vi "Ex2_PagWeb.vi"(0 "WebBrowser":refnum<k7>(container), 8 "stop":bool, 11 "Web Page URL":string="http://") -> (3 "Web Page Title":string)   [LabVIEW 2020]
doc: "This example uses the Microsoft WebBrowser ActiveX control. It demonstrates how to register an ActiveX event callback and extract event data."
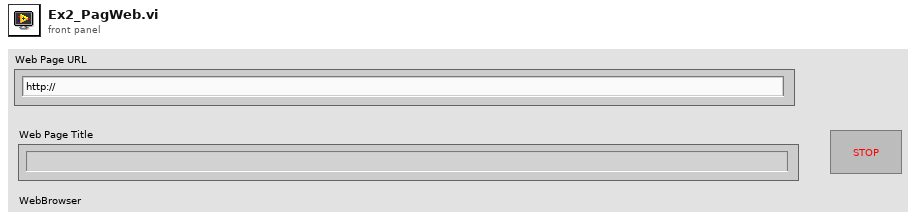
[diagram p1: front panel]
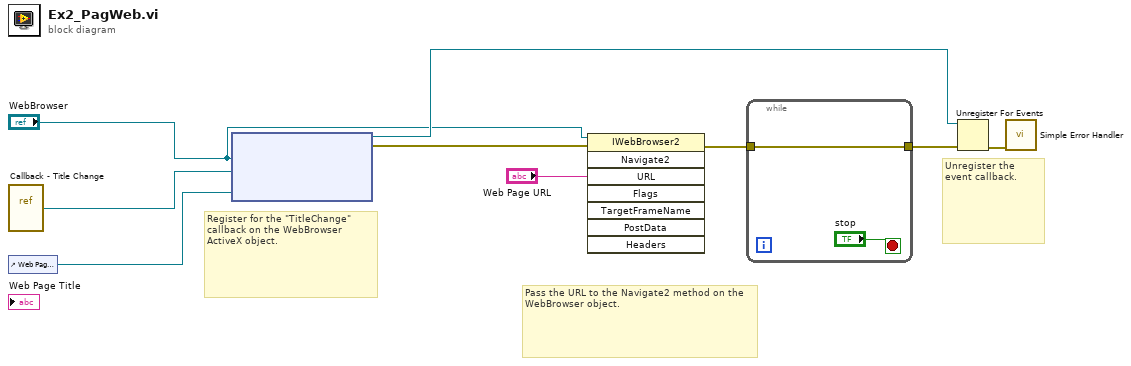
[diagram p0: block diagram]
diagram:
  # "Pass the URL to the Navigate2 method on the WebBrowser object."
  # "Unregister the event callback."
  # "Register for the \"TitleChange\" callback on the WebBrowser ActiveX object."
  n1 = vi-ref "Callback - Title Change.vi"() -> ("vi reference"=w8:refnum<vi>)
  n2 = control-ref of="Web Page Title"() -> (w9:refnum<vi>)
  n3 = node("WebBrowser", w8, w9) -> (w6:refnum<k27>, w4:errorcluster)  [unwired: 2 in]
  n4 = invoke class="IWebBrowser2" method="Navigate2"(reference="WebBrowser", error in=w4, "URL"="Web Page URL") -> (error out=w2:errorcluster)  [unwired: 5 in, 7 out]
  n5 = while {
    tunnel: [w10] -> w1
    tunnel: w2 -> [w10]
    stop <- "stop" stop-if-true
  }
  n6 = Unregister For Events(event registration refnum=w6, error in=w1) -> (error out=w7:errorcluster)
  n7 = call <vilib>:"Simple Error Handler.vi"("error in (no error)"=w7) -> ()  [unwired: 4 in, 5 out]
